vi "Write separate compiled code.vi"(8 "error in (no error)":errorcluster, 10 "separate compiled code":bool, 11 "set source separate in":refnum<class "set source separate.lvclass">) -> (0 "error out":errorcluster, 3 "set source separate out":refnum<class "set source separate.lvclass">)   [LabVIEW 2013, in "set source separate.lvclass"]
uses:
  set source separate.lvclass
  set source separate.lvclass/set source separate.ctl
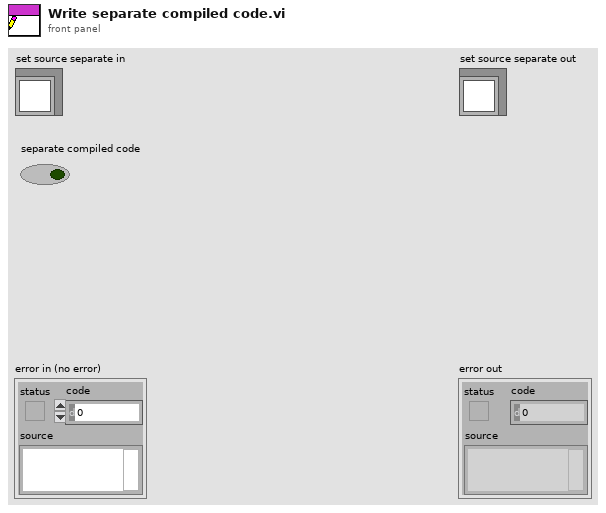
[diagram p1: front panel]
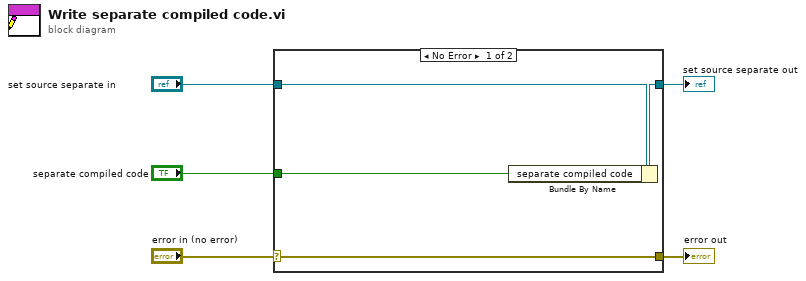
[diagram p0: block diagram]
diagram:
  n1 = case shown="No Error" "error in (no error)" {
    selector: "error in (no error)" -> [w9 w10]
    tunnel: [w9 w10] -> w4
    tunnel: [w7 w11] -> w2
    tunnel: "set source separate in" -> [w8 w11]
    tunnel: "separate compiled code" -> [w6 _]
    frame No Error {
      n2 = Bundle By Name(cluster=w8, "separate compiled code"=w6) -> (w7:refnum<class "set source separate.lvclass">)
    }
    frame Error {
    }
  }
  "error out" <- w4
  "set source separate out" <- w2
